vi "Get Temperature (Celsius).vi"(8 "Error In":errorcluster, 11 "Dual Mode Thermometer in":refnum<class "Dual Mode Thermometer.lvclass">) -> (0 "Error Out":errorcluster, 2 "Temperature (Celsius)":dbl, 3 "Dual Mode Thermometer out":refnum<class "Dual Mode Thermometer.lvclass">)   [LabVIEW 2014, in "Porting from XControls - Dual Mode Thermometer.lvlib" / "Dual Mode Thermometer.lvclass"]
doc: "Copyright (c) 2016 Sze Howe Koh\nThis code is licensed under the MIT license"
uses:
  Dual Mode Thermometer.lvclass
  Dual Mode Thermometer.lvclass/Dual Mode Thermometer.ctl
  src/LabVIEW/Qwt/QwtAbstractSlider/QwtAbstractSlider.lvclass
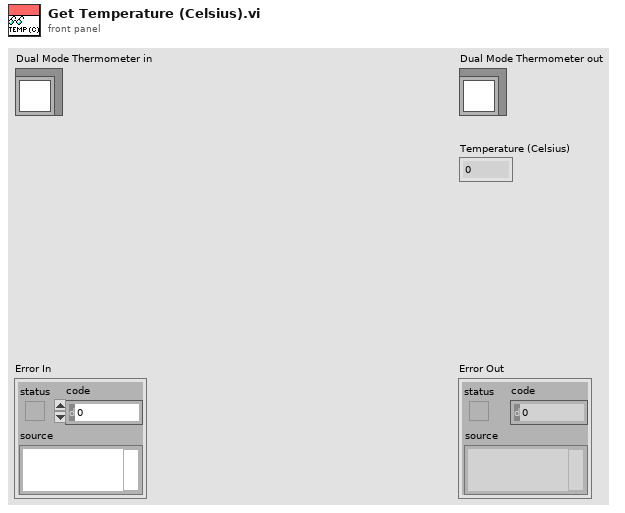
[diagram p1: front panel]
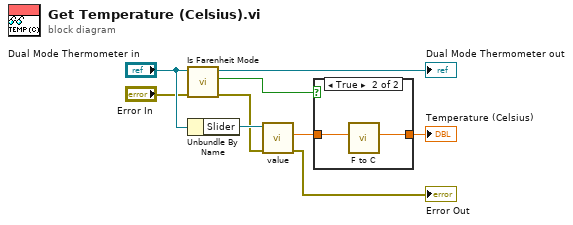
[diagram p0: block diagram]
diagram:
  n1 = call "Is Farenheit Mode.vi"("Error In"="Error In", "Dual Mode Thermometer In"="Dual Mode Thermometer in") -> ("Error Out"=w2:errorcluster, "Farenheit Mode"=w1:bool, "Dual Mode Thermometer out"=→"Dual Mode Thermometer out":refnum<class "Dual Mode Thermometer.lvclass">)  [unwired: 7 in]
  n2 = Unbundle By Name("Dual Mode Thermometer in") -> ("Slider"=w9:refnum<class "QwtSlider.lvclass">)
  n3 = call "value.vi"("Error In"=w2, "QwtAbstractSlider In"=w9) -> ("Error Out"=→"Error Out":errorcluster, "Value"=w7:dbl)  [unwired: 7 in, 1 out]
  n4 = case shown="True" w1 {
    tunnel: w7 -> [w10 w12]
    tunnel: [w10 w11] -> w6
    frame False {
    }
    frame True {
      n5 = call "F to C.vi"("Value [°F]"=w12) -> ("Value [°C]"=w11:dbl)  [unwired: 10 in]
    }
  }
  "Temperature (Celsius)" <- w6
